vi "DEPP Set Test.vi"() -> ()   [LabVIEW 2011, in "LVH-Adept.lvlib"]
uses:
  LVH-Adept.lvlib
  Private/DMGR/DMGR.lvlib
  Private/DEPP/DEPP.lvlib
panel:
  out "Data 2":u8[](array[numeric])
  in  "Addresses 2":u8[](array[numeric])=[0, 1, 2, 3, 4, 5, 6]
  in  "Data":u8[](array[numeric])=[0, 22, 44, 66]
  in  "Addresses":u8[](array[numeric])=[0, 2, 4, 6]
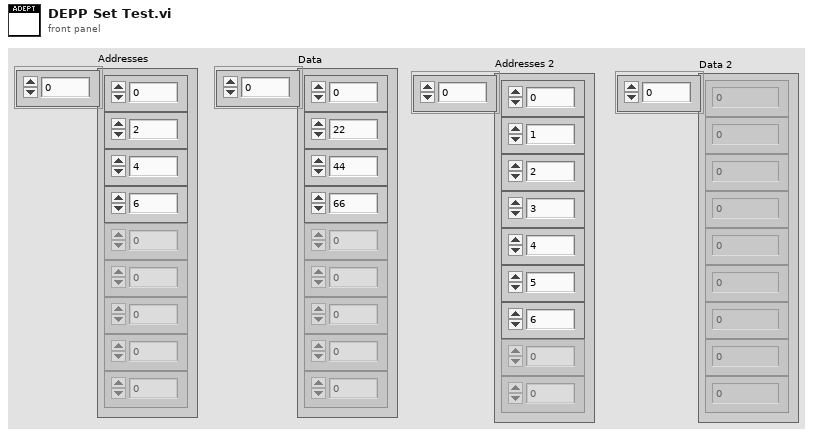
[diagram p1: front panel]
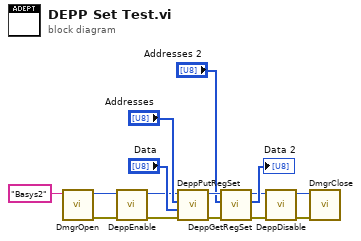
[diagram p0: block diagram]
diagram:
  n1 = call "DmgrOpen.vi"("Device Name"="Basys2") -> ("Error Out"=w3:errorcluster, "Device Handle"=w4:u32)  [unwired: 9 in]
  n2 = call "DeppEnable.vi"("Error In"=w3, "Device Handle"=w4) -> ("Error Out"=w1:errorcluster, "Device Handle"=w2:u32)  [unwired: 8 in]
  n3 = call "DeppPutRegSet.vi"("Error In"=w1, "Data"="Data", "Addresses"="Addresses", "Device Handle"=w2) -> ("Error Out"=w14:errorcluster, "Device Handle"=w15:u32)  [unwired: 6 in]
  n4 = call "DeppGetRegSet.vi"("Error In"=w14, "Addresses"="Addresses 2", "Device Handle"=w15) -> ("Error Out"=w5:errorcluster, "Data"=→"Data 2":u8[], "Device Handle"=w6:u32)  [unwired: 6 in]
  n5 = call "DeppDisable.vi"("Error In"=w5, "Device Handle"=w6) -> ("Error Out"=w8:errorcluster, "Device Handle"=w7:u32)  [unwired: 8 in]
  n6 = call "DmgrClose.vi"("Error In"=w8, "hif"=w7) -> ()  [unwired: 9 in, 1 out]
